vi "Test Sort 2D Arr String.vi"() -> ()   [LabVIEW 2014]
panel:
  out "sorted array":T1(array[cluster])
  out "Array":T1(array[cluster])
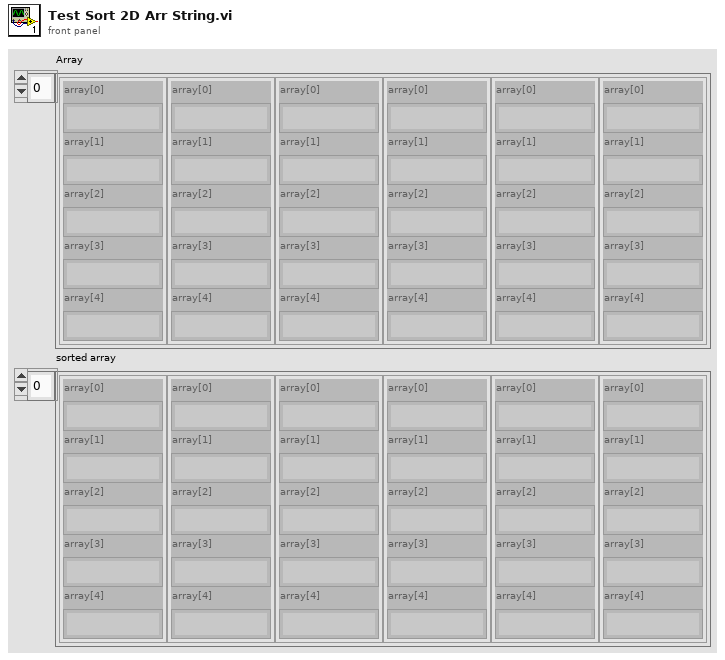
[diagram p1: front panel]
types:
  T1 = cluster{"array[0]":string, "array[1]":string, "array[2]":string, "array[3]":string, "array[4]":string}[]
  T2 = cluster{"array[0]":string, "array[1]":string, "array[2]":string, "array[3]":string, "array[4]":string}
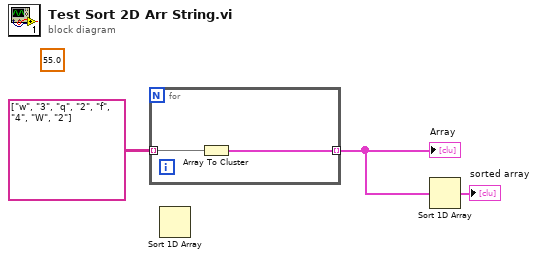
[diagram p0: block diagram]
diagram:
  (unwired) 55.0
  n1 = for {
    tunnel: string[][] [["w", "3"], ["q", "2"], ["f", "4"], ["W", "2"]] ("array") -> [w5] mode=indexing
    tunnel: [w4] -> w3 mode=indexing
    n2 = Array To Cluster(array=w5) -> (cluster=w4:T2)
  }
  "Array" <- w3
  n3 = Sort 1D Array() -> ()  [unwired: 1 in, 1 out]
  n4 = Sort 1D Array(array=w3) -> (sorted array=→"sorted array":T1)
